vi "SerializeAttributes.vi"(7 "MsgSerializer":refnum<class "MsgSerializer.lvclass">, 10 "attribute name":string, 11 "variant attribute":variant) -> (3 "Serialized Message":string)   [LabVIEW 2020, in "Caraya.lvlib" / "Test Report.JUnit.lvclass"]
uses:
  Test Report.JUnit.lvclass
  MsgSerializer/MsgSerializer.lvclass
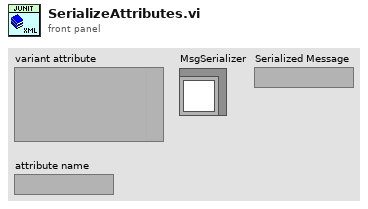
[diagram p1: front panel]
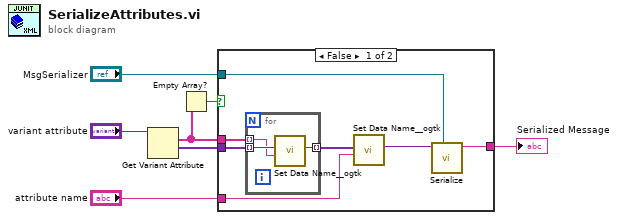
[diagram p0: block diagram]
diagram:
  n1 = Get Variant Attribute(Variant="variant attribute") -> (names=w6:string[], values=w4:variant[])  [unwired: 3 in, 2 out]
  n2 = Empty Array?(array=w6) -> (empty?=w7:bool)
  n3 = case shown="False" w7 {
    tunnel: [w14 _] -> w2
    tunnel: w4 -> [w13 _]
    tunnel: "attribute name" -> [w10 _]
    tunnel: w6 -> [w9 _]
    tunnel: "MsgSerializer" -> [w8 _]
    frame False {
      n4 = for {
        tunnel: w9 -> [w16] mode=indexing
        tunnel: w13 -> [w17] mode=indexing
        tunnel: [w15] -> w12 mode=indexing
        n5 = call <userlib>:"Set Data Name__ogtk.vi"("Data Name"=w16, "Data"=w17) -> ("Renamed Data"=w15:variant)  [unwired: 8 in, 1 out]
      }
      n6 = call <userlib>:"Set Data Name__ogtk.vi"("Data Name"=w10, "Data"=w12) -> ("Renamed Data"=w11:variant)  [unwired: 8 in, 1 out]
      n7 = call-dynamic "Serialize.vi"("MsgSerializer"=w8, "Value"=w11) -> ("Serialized Message"=w14:string)  [unwired: 8 in, 1 out]
    }
    frame True {
    }
  }
  "Serialized Message" <- w2
